vi "Cooling Tower Experiment v1_a.vi"() -> ()   [LabVIEW 2019]
uses:
  <vilib>/Utility/file.llb/Write To Spreadsheet File (DBL).vi
panel:
  in  "Clear Graph":bool
  in  "Record":bool
  in  "Shut off":bool
  out "Resevoir Temp":dbl format="%.1g"
  out "Elapsed Time (min)":dbl caption="Elapsed Time (s)" format="%.2g"
  out "Inlet Dry Bulb Temp":dbl format="%.1g"
  out "Inlet Wet Bulb Temp":dbl format="%.1g"
  out "Outlet Wet Bulb Temp":dbl format="%.1g"
  out "Outlet Dry Bulb Temp":dbl format="%.1g"
  out "Inlet Water Temp":dbl format="%.1g"
  out "Outlet Water Temp":dbl format="%.1g"
  in  "Plot and Save":bool
  in  "Continuous Plotting?":bool
  out "Waveform Chart":T1(graph)
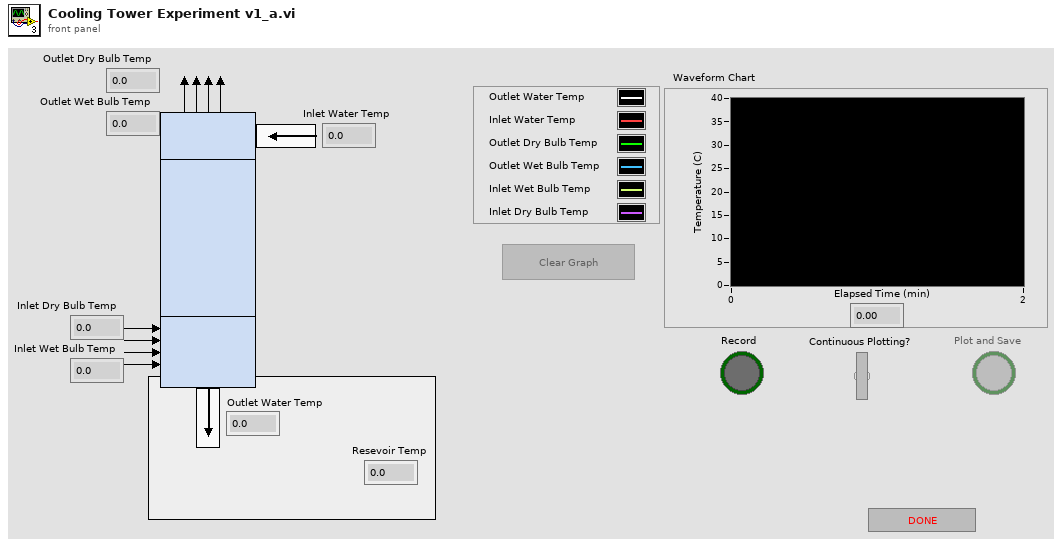
[diagram p1: front panel]
types:
  T1 = cluster{"Outlet Water Temp":dbl, "Inlet Water Temp":dbl, "Outlet Dry Bulb Temp":dbl, "Outlet Wet Bulb Temp":dbl, "Inlet Wet Bulb Temp":dbl, "Inlet Dry Bulb Temp ":dbl, "Resevoir Temp":dbl}
  T2 = cluster{"Outlet Water Temp":dbl, "Inlet Water Temp":dbl, "Outlet Dry Bulb Temp":dbl, "Outlet Wet Bulb Temp":dbl, "Inlet Wet Bulb Temp":dbl, "Inlet Dry Bulb Temp ":dbl, "Resevoir Temp":dbl}[]
  T3 = enum8{"Enabled", "Disabled", "Disabled and Grayed Out"}
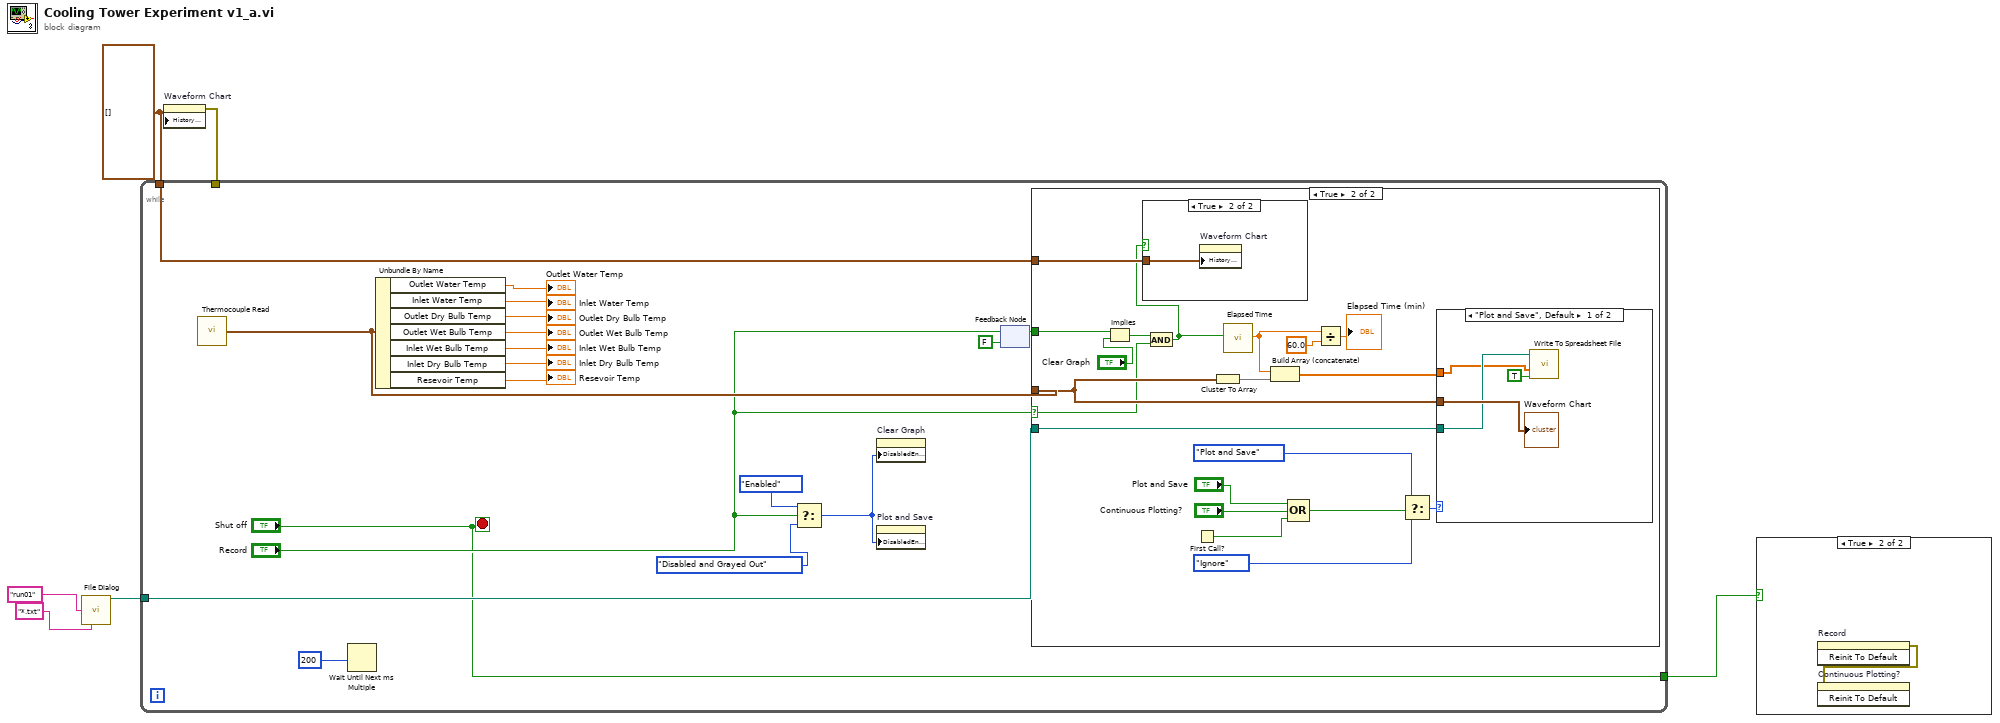
[diagram p0: block diagram]
diagram:
  w2 = T2 [] ("History Data")
  n1 = call "File Dialog"("default name"="run01", "pattern (all files)"="*.txt") -> ("selected path"=w3:path)  [unwired: 10 in, 3 out]
  n2 = property on="Waveform Chart" class="WFChart (strict)"("History Data"=w2) -> (error out=w6:errorcluster)  [unwired: 2 in, 1 out]
  n3 = while {
    tunnel: w6 -> [_]
    tunnel: w3 -> [w17]
    tunnel: w2 -> [w13]
    tunnel: ["Shut off"] -> w1
    stop <- "Shut off" stop-if-true
    n4 = call "Thermocouple Read.vi"() -> ("Cluster"=w18:T1)  [unwired: 1 in]
    n5 = Wait Until Next ms Multiple(millisecond multiple=u32 200) -> ()  [unwired: 1 out]
    n6 = Unbundle By Name(w18) -> ("Outlet Water Temp"=→"Outlet Water Temp":dbl, "Inlet Water Temp"=→"Inlet Water Temp":dbl, "Outlet Dry Bulb Temp"=→"Outlet Dry Bulb Temp":dbl, "Outlet Wet Bulb Temp"=→"Outlet Wet Bulb Temp":dbl, "Inlet Wet Bulb Temp"=→"Inlet Wet Bulb Temp":dbl, "Inlet Dry Bulb Temp"=→"Inlet Dry Bulb Temp":dbl, "Resevoir Temp"=→"Resevoir Temp":dbl)
    n7 = Select(t=T3."Enabled" ("Disabled"), s="Record", f=T3."Disabled and Grayed Out" ("Disabled")) -> (s? t:f=w12:T3)
    n8 = property on="Clear Graph" class="Bool"("DisabledEnum"=w12) -> ()  [unwired: 2 in, 2 out]
    n9 = property on="Plot and Save" class="Bool"("DisabledEnum"=w12) -> ()  [unwired: 2 in, 2 out]
    n10 = feedback-in #1("Record") -> ()
    n11 = feedback #1(FALSE ("Record")) -> (w10:bool)
    n12 = case shown="True" "Record" {
      selector: "Record" -> [_ w28]
      tunnel: w18 -> [_ w38]
      tunnel: w17 -> [_ w36]
      tunnel: w13 -> [_ w30]
      tunnel: w10 -> [_ w26]
      frame False {
      }
      frame True {
        n13 = Implies(1:"Clear Graph", 2:w26) -> (0:w27:bool)
        n14 = And(x=w27, y=w28) -> (x .and. y?=w29:bool)
        n15 = case shown="True" w29 {
          tunnel: w30 -> [_ w45]
          frame False {
          }
          frame True {
            n16 = property on="Waveform Chart" class="WFChart (strict)"("History Data"=w45) -> ()  [unwired: 2 in, 2 out]
          }
        }
        n17 = First Call?() -> (First Call?: T/F=w37:bool)
        n18 = Cluster To Array(cluster=w38) -> (array=w33:dbl[])
        n19 = call "Elapsed Time"("Reset"=w29) -> ("Elapsed Time (s)"=w34:dbl)  [unwired: 11 in, 7 out]
        n20 = Build Array (concatenate)(w34, w33) -> (w35:dbl[])
        n21 = Compound Arithmetic op=OR("Plot and Save", "Continuous Plotting?", w37) -> (w41:bool)
        n22 = Divide(x=w34, y=60.0) -> (x/y=→"Elapsed Time (min)":dbl)
        n23 = Select(t=enum16{"Plot and Save", "Ignore"}."Plot and Save", s=w41, f=enum16{"Plot and Save", "Ignore"}."Ignore") -> (s? t:f=w44:enum16{"Plot and Save", "Ignore"})
        n24 = case shown="\"Plot and Save\", Default" w44 {
          tunnel: w38 -> [w49 _]
          tunnel: w36 -> [w48 _]
          tunnel: w35 -> [w46 _]
          frame "Plot and Save", Default {
            n25 = call-poly <vilib>:"Write To Spreadsheet File.vi"("append to file? (new file:F)"=TRUE, "1D data"=w46, "file path (dialog if empty)"=w48) -> ()  [unwired: 5 in, 1 out]
            "Waveform Chart" <- w49
          }
          frame "Ignore" {
          }
        }
      }
    }
  }
  n26 = case shown="True" w1 {
    frame False {
    }
    frame True {
      n27 = invoke on="Record" class="Bool (strict)" method="Reinit To Default"() -> (error out=w50:errorcluster)  [unwired: 3 in, 2 out]
      n28 = invoke on="Continuous Plotting?" class="Bool (strict)" method="Reinit To Default"(error in=w50) -> ()  [unwired: 2 in, 3 out]
    }
  }
